vi "Initialize Transfer Group Parameters.vi"(8 "error in (no error)":errorcluster, 10 "Transfer Groups Configurations":T1[](array[typedef]) {"Transfers"."channels"."string offset" format="%d bytes"}, 11 "GE Reflective Memory Transceiver in":refnum<class "GE Reflective Memory Transceiver.lvclass">) -> (0 "error out":errorcluster, 3 "GE Reflective Memory Transceiver out":refnum<class "GE Reflective Memory Transceiver.lvclass">)   [LabVIEW 2017, in "GE Reflective Memory Transceiver.lvlib" / "GE Reflective Memory Transceiver.lvclass"]
uses:
  GE Reflective Memory Transceiver.lvclass
  Builds/Data Sharing Framework/Current/Core/DSF Core.lvlibp/Typedefs/DSF Engine Transfer Group Configuration.ctl
  Builds/Data Sharing Framework/Current/Core/DSF Core.lvlibp/Typedefs/DSF Direction.ctl
  Builds/Data Sharing Framework/Current/Core/DSF Core.lvlibp/Typedefs/DSF Timing Info.ctl
  Builds/Data Sharing Framework/Current/Core/DSF Core.lvlibp/Typedefs/DSF Settings Info.ctl
  Builds/Data Sharing Framework/Current/Core/DSF Core.lvlibp/Typedefs/DSF Engine Transfer Configuration.ctl
  Builds/Data Sharing Framework/Current/Core/DSF Core.lvlibp/Typedefs/DSF Byte Order.ctl
  Builds/Data Sharing Framework/Current/Core/DSF Core.lvlibp/Typedefs/DSF Engine Channel Configuration.ctl
  Builds/Data Sharing Framework/Current/Core/DSF Core.lvlibp/Typedefs/DSF Data Type.ctl
  Builds/Data Sharing Framework/Current/Core/DSF Core.lvlibp/Typedefs/DSF Timeout Behavior.ctl
  Transfer Group Parameters.ctl
  <vilib>/NI/GE Reflective Memory Driver/Typedefs/GE 5565PIORC.Typedef.DMA Transfer Spec.ctl
  <vilib>/NI/GE Reflective Memory Driver/Typedefs/GE 5565PIORC.Typedef.DMA Block Descriptor.ctl
  <vilib>/NI/GE Reflective Memory Driver/Typedefs/GE 5565PIORC.Typedef.DMA Block Descriptor Params.ctl
  GE Reflective Memory Transceiver.lvclass/GE Reflective Memory Transceiver.ctl
  <vilib>/NI/GE Reflective Memory Driver/GE 5565PIORC.lvclass/GE 5565PIORC.ctl
  <vilib>/NI/GE Reflective Memory Driver/Methods/GE 5565PIORC.DMA.Create Transfer (Block).vi
  <vilib>/NI/GE Reflective Memory Driver/Methods/GE 5565PIORC.DMA.Create Transfer (Scatter-Gather).vi
  <vilib>/NI/GE Reflective Memory Driver/Methods/GE 5565PIORC.DMA.Size.vi
  <vilib>/NI/GE Reflective Memory Driver/Methods/GE 5565PIORC.Round Up to Nearest 8.vi
  <vilib>/NI/GE Reflective Memory Driver/Methods/GE 5565PIORC.Round Up to Nearest 16.vi
  <vilib>/NI/GE Reflective Memory Driver/GE 5565PIORC.lvclass
  Builds/Data Sharing Framework/Current/Core/DSF Core.lvlibp
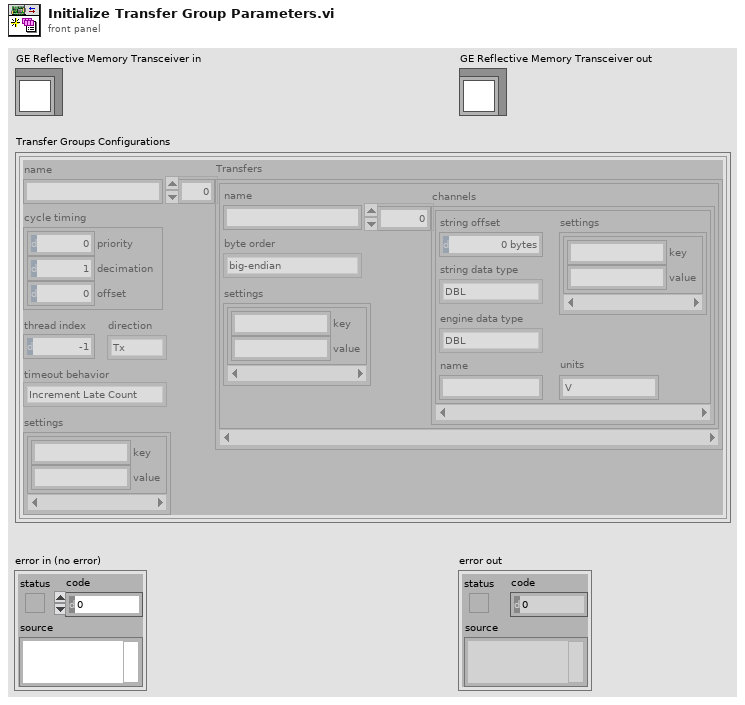
[diagram p1: front panel]
types:
  T1 = typedef "DSF Core.lvlibp/DSF Engine Transfer Group Configuration.ctl" = cluster{"name":string, "direction":T2, "cycle timing":T3, "thread index":i32, "settings":T4, "Transfers":T5[], "timeout behavior":T9}
  T2 = typedef "DSF Core.lvlibp/DSF Direction.ctl" = enum8{"Tx", "Rx"}
  T3 = typedef "DSF Core.lvlibp/DSF Timing Info.ctl" = cluster{"priority":u64, "decimation":u64, "offset":u64}
  T4 = typedef "DSF Core.lvlibp/DSF Settings Info.ctl" = cluster{"key":string, "value":string}[]
  T5 = typedef "DSF Core.lvlibp/DSF Engine Transfer Configuration.ctl" = cluster{"name":string, "byte order":T6, "settings":T4, "channels":T7[]}
  T6 = typedef "DSF Core.lvlibp/DSF Byte Order.ctl" = enum8{"big-endian", "little-endian"}
  T7 = typedef "DSF Core.lvlibp/DSF Engine Channel Configuration.ctl" = cluster{"string offset":u64, "string data type":T8, "engine data type":T8, "name":string, "settings":T4, "units":string}
  T8 = typedef "DSF Core.lvlibp/DSF Data Type.ctl" = enum8{"Bool", "SGL", "DBL", "I8", "I16", "I32", "I64", "U8", "U16", "U32", "U64"}
  T9 = typedef "DSF Core.lvlibp/DSF Timeout Behavior.ctl" = enum8{"Increment Late Count", "Throw Error"}
  T10 = typedef "GE Reflective Memory Transceiver.lvlib/GE Reflective Memory Transceiver.lvclass/Transfer Group Parameters.ctl" = cluster{"DMA Transfer Specs":T11[]}
  T11 = typedef "GE 5565PIORC.lvclass/GE 5565PIORC.Typedef.DMA Transfer Spec.ctl" = cluster{"RFM offset":u32, "Block Descriptors":T12[]}
  T12 = typedef "GE 5565PIORC.lvclass/GE 5565PIORC.Typedef.DMA Block Descriptor.ctl" = cluster{"descriptor ptr (VISA)":u32, "descriptor ptr (RFM)":u32, "descriptor size":u32, "descriptor params":T13}
  T13 = typedef "GE 5565PIORC.lvclass/GE 5565PIORC.Typedef.DMA Block Descriptor Params.ctl" = cluster{"data ptr (lower)":u32, "data ptr (upper)":u32, "data size":u32, "next descriptor ptr":u32}
  T14 = typedef "GE Reflective Memory Transceiver.lvlib/GE Reflective Memory Transceiver.lvclass/Transfer Parameters.ctl" = cluster{"offset":u32, "size":u32}
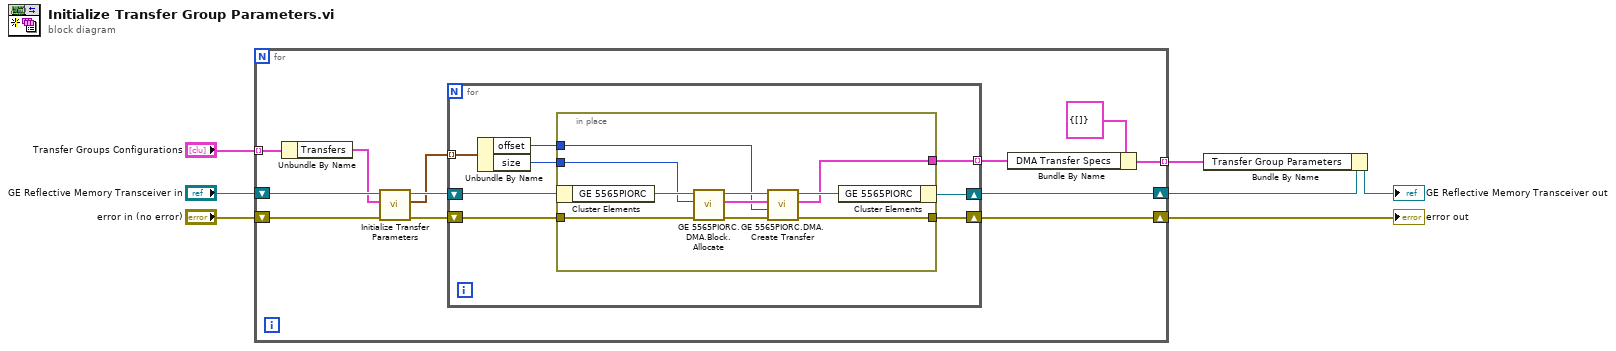
[diagram p0: block diagram]
diagram:
  n1 = for {
    tunnel: "Transfer Groups Configurations" -> [w9] mode=indexing
    shift-right: [w12] -> w3
    shift-left: "GE Reflective Memory Transceiver in" -> [w16]
    shift-right: [w11] -> w4
    shift-left: "error in (no error)" -> [w17]
    tunnel: [w18] -> w1 mode=indexing
    n2 = Unbundle By Name(w9) -> ("Transfers"=w8:T5[])
    n3 = call "Initialize Transfer Parameters.vi"("error in (no error)"=w17, "Transfer Configurations"=w8, "DSF GE Reflective Memory Transceiver in"=w16) -> ("error out"=w15:errorcluster, "Transfers Parameters"=w13:T14[], "DSF GE Reflective Memory Transceiver out"=w14:refnum<class "GE Reflective Memory Transceiver.lvclass">)  [unwired: 6 in]
    n4 = for {
      tunnel: w13 -> [w25] mode=indexing
      shift-right: [w21] -> w11
      shift-left: w15 -> [w27]
      tunnel: [w22] -> w10 mode=indexing
      shift-right: [w20] -> w12
      shift-left: w14 -> [w26]
      n5 = Unbundle By Name(w25) -> ("offset"=w23:u32, "size"=w24:u32)
      n6 = in-place {
        in-place-border: [w36] -> w21
        in-place-border: [w30] -> w22
        in-place-border: w27 -> [w32]
        in-place-border: w24 -> [w31]
        in-place-border: w23 -> [w28]
        n7 = in-place-cluster #1(w26) -> ("GE 5565PIORC"=w34:refnum<class "GE 5565PIORC.lvclass">)
        n8 = call <vilib>:"GE 5565PIORC.DMA.Block.Allocate.vi"("error in (no error)"=w32, "size in bytes"=w31, "GE 5565PIORC in"=w34) -> ("error out"=w37:errorcluster, "Block Descriptor"=w29:T12, "GE 5565PIORC out"=w35:refnum<class "GE 5565PIORC.lvclass">)  [unwired: 6 in]
        n9 = call-poly <vilib>:"GE 5565PIORC.DMA.Create Transfer.vi"("error in (no error)"=w37, "RFM offset"=w28, "Block Descriptor"=w29, "GE 5565PIORC in"=w35) -> ("error out"=w36:errorcluster, "DMA Transfer Spec"=w30:T11, "GE 5565PIORC out"=w33:refnum<class "GE 5565PIORC.lvclass">)  [unwired: 4 in, 1 out]
        n10 = in-place-cluster #1("GE 5565PIORC"=w33) -> (w20:refnum<class "GE Reflective Memory Transceiver.lvclass">)
      }
    }
    n11 = Bundle By Name(cluster=T10 {"DMA Transfer Specs"=[]} ("Transfer Group Parameters"), "DMA Transfer Specs"=w10) -> (w18:T10)
  }
  "error out" <- w4
  n12 = Bundle By Name(cluster=w3, "Transfer Group Parameters"=w1) -> (→"GE Reflective Memory Transceiver out":refnum<class "GE Reflective Memory Transceiver.lvclass">)
